vi "GetQuestion.vi"(7 "LabVIEW Web Service Request":refnum<class "Web Request.lvclass">) -> ()   [LabVIEW 2014]
uses:
  <vilib>/wsapi/Web Request.lvclass
  Coding Platform.lvlib
panel:
  # "Use the Web Service Request input terminal to call the VIs on the Web Services palette. Do not remove it from the connector pane unless you don't need access to the palette."
  # "Each additional control wired to the connector pane will be available as an input in the URL. To include an indicator in terminal-mode output (the default setting), it must also be wired to the connector pane."
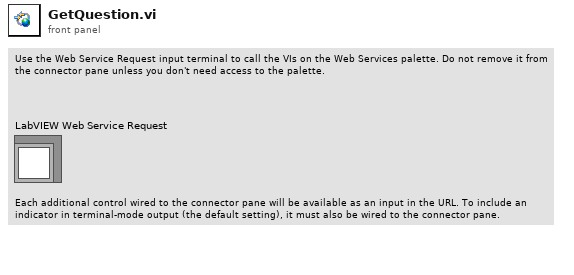
[diagram p1: front panel]
types:
  T1 = typedef "Coding Platform.lvlib/Question Response.ctl" = cluster{"QuestionTitle":string, "Question":string, "Description":string}
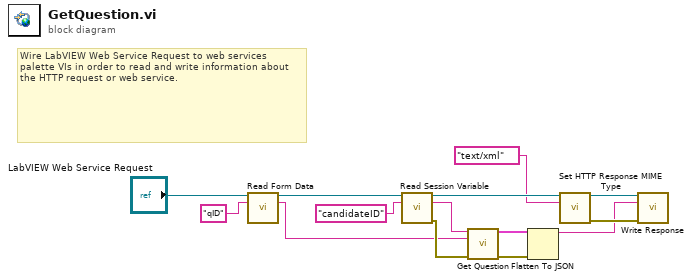
[diagram p0: block diagram]
diagram:
  # "Wire LabVIEW Web Service Request to web services palette VIs in order to read and write information about the HTTP request or web service."
  n1 = call <vilib>:"Read Form Data.vi"("LabVIEW Web Service Request"="LabVIEW Web Service Request", "key"="qID") -> ("LabVIEW Web Service Request out"=w2:refnum<class "Web Request.lvclass">, "value"=w1:string)  [unwired: 10 in, 2 out]
  n2 = call <vilib>:"Read Session Variable.vi"("LabVIEW Web Service Request"=w2, "key"="candidateID") -> ("LabVIEW Web Service Request out"=w12:refnum<class "Web Request.lvclass">, "value"=w5:string, "error out"=w14:errorcluster)  [unwired: 11 in]
  n3 = call "Get Question.vi"("Candidate ID"=w5, "Question_ID"=w1, "error in (no error)"=w14) -> ("Cluster"=w13:T1, "error out"=w11:errorcluster)  [unwired: 11 in]
  n4 = Flatten To JSON(anything=w13, error in (no error)=w11) -> (JSON string=w7:string)  [unwired: 1 in, 1 out]
  n5 = call <vilib>:"Set HTTP Response MIME Type.vi"("LabVIEW Web Service Request"=w12, "MIME type (text/html)"="text/xml") -> ("LabVIEW Web Service Request out"=w10:refnum<class "Web Request.lvclass">, "error out"=w9:errorcluster)  [unwired: 12 in]
  n6 = call <vilib>:"Write Response.vi"("LabVIEW Web Service Request"=w10, "response string"=w7, "error in (no error)"=w9) -> ()  [unwired: 11 in, 2 out]
